vi "TranslateHom2D.vi"(0 "points":dbl[][](array[numeric])=[[0.0, 1.0, 79.632, 72.629, 0.0, 0.0, 1.0], [0.0, 2.0, 79.632, 159.629, 0.0, 0.0, 1.0], [0.0, 3.0, 90.632, 83.629, 0.0, 0.0, 1.0], [0.0, 4.0, 93.632, 156.629, 0.0, 0.0, 1.0], [0.0, 5.0, 192.632, 85.129, 0.0, 0.0, 1.0], [0.0, 6.0, 202.632, 159.629, 0.0, 0.0, 1.0], [0.0, 7.0, 208.632, 147.129, 0.0, 0.0, 1.0], [0.0, 8.0, 229.132, 68.129, 0.0, 0.0, 1.0], [0.0, 0.0, 0.0, 0.0, 0.0, 0.0, 0.0]], 1 "Camera":dbl[](array[numeric]), 2 "Robot":dbl[](array[numeric]), 5 "Steps":dbl[][](array[numeric])=[[0.0, 1.0, 79.632, 72.629, 0.0, 0.0, 1.0], [0.0, 2.0, 79.632, 159.629, 0.0, 0.0, 1.0], [0.0, 3.0, 90.632, 83.629, 0.0, 0.0, 1.0], [0.0, 4.0, 93.632, 156.629, 0.0, 0.0, 1.0], [0.0, 5.0, 192.632, 85.129, 0.0, 0.0, 1.0], [0.0, 6.0, 202.632, 159.629, 0.0, 0.0, 1.0], [0.0, 7.0, 208.632, 147.129, 0.0, 0.0, 1.0], [0.0, 8.0, 229.132, 68.129, 0.0, 0.0, 1.0], [0.0, 0.0, 0.0, 0.0, 0.0, 0.0, 0.0]], 9 "Angle":dbl, 11 "错误输入（无错误）":errorcluster, 12 "RealCamera":cluster{"X":dbl, "Y":dbl} {"X" format="%#_13g"}) -> (4 "ListPoints":dbl[][](array[numeric]), 6 "StringPoints":string[][](array[string]), 15 "错误输出":errorcluster)   [LabVIEW 2016]
uses:
  X86/halcondotnet.dll
panel:
  out "数组 2":dbl[](array[numeric])
  out "数组":dbl[](array[numeric])
  out "x-y":dbl
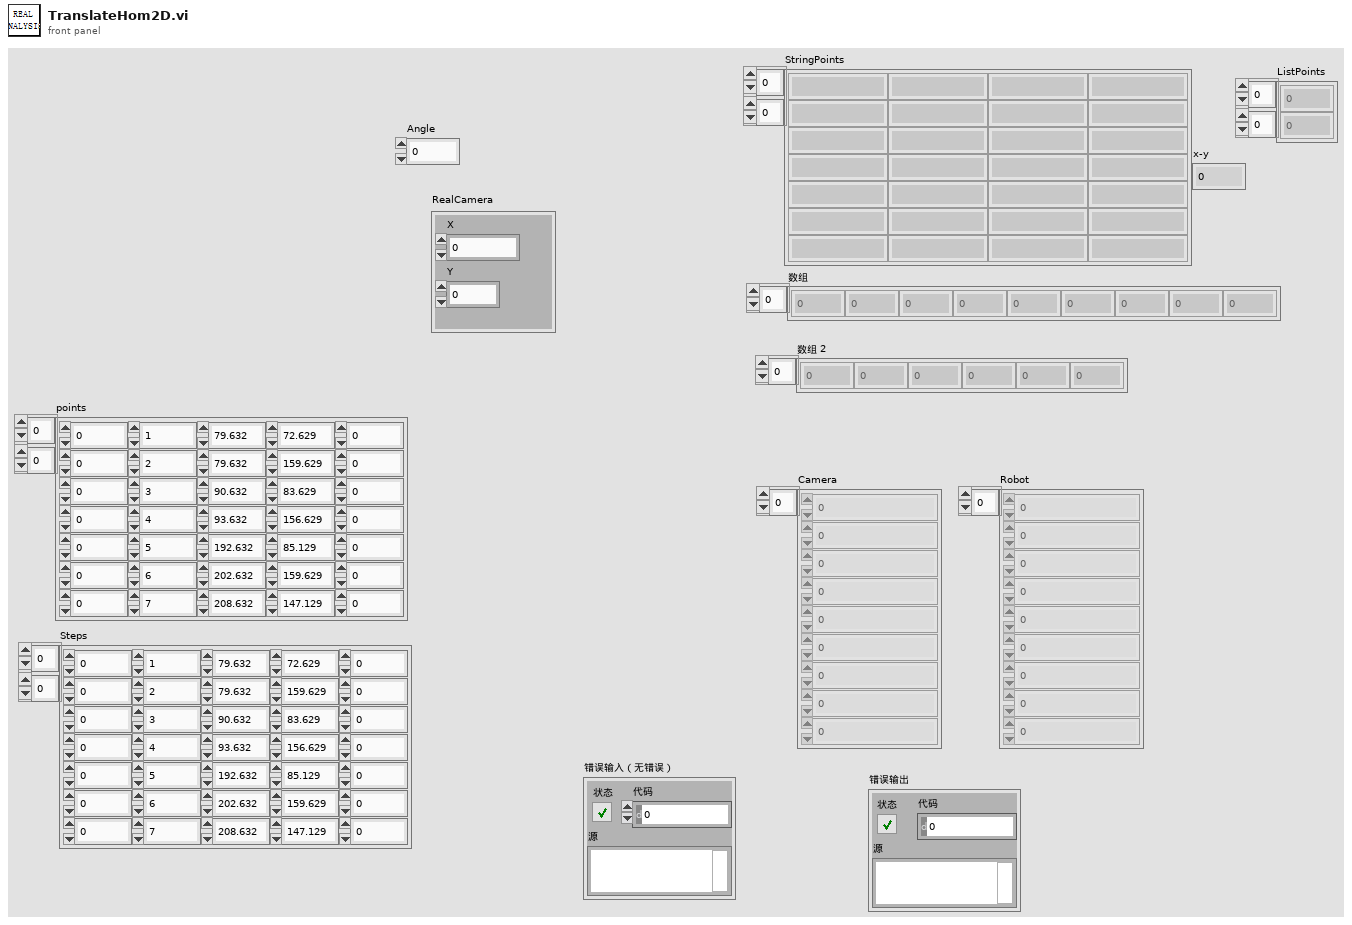
[diagram p1: front panel]
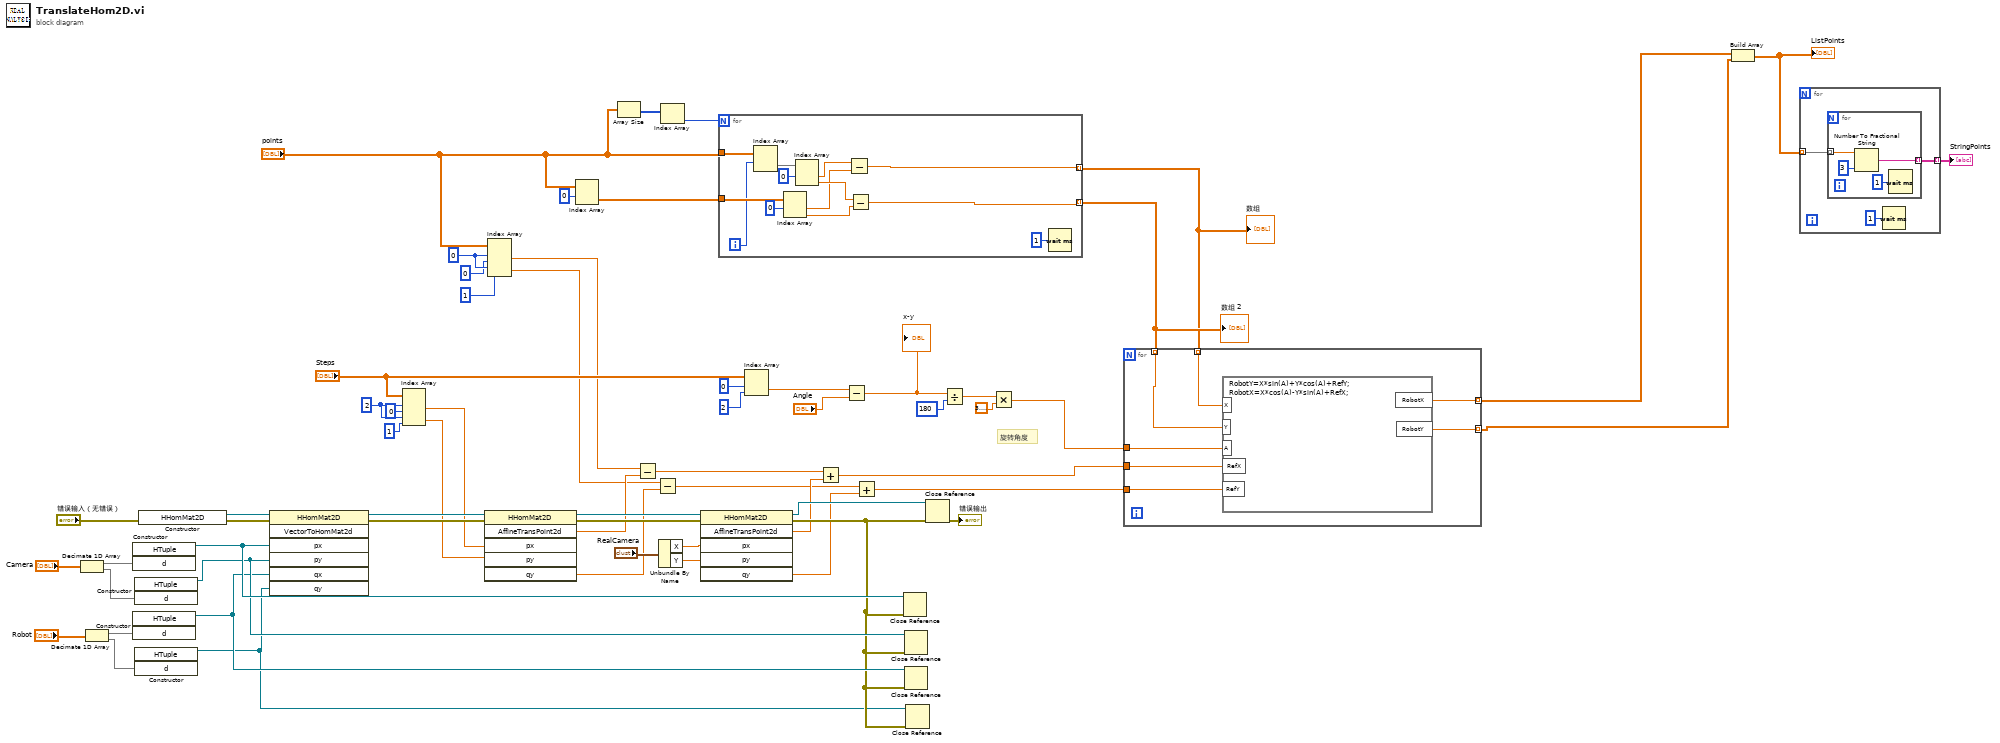
[diagram p0: block diagram]
diagram:
  w19 = 0 ("索引 (行)")
  w25 = 2 ("索引 (行)")
  # "旋转角度"
  n1 = Decimate 1D Array("Camera") -> (w60:dbl[], w59:dbl[])
  n2 = Decimate 1D Array("Robot") -> (w58:dbl[], w57:dbl[])
  n3 = constructor class="HTuple"("d"=w60) -> (reference out=w50:refnum<k24>)  [unwired: 3 in, 3 out]
  n4 = constructor class="HTuple"("d"=w58) -> (reference out=w48:refnum<k24>)  [unwired: 3 in, 3 out]
  n5 = constructor class="HTuple"("d"=w59) -> (reference out=w49:refnum<k24>)  [unwired: 3 in, 3 out]
  n6 = constructor class="HTuple"("d"=w57) -> (reference out=w46:refnum<k24>)  [unwired: 3 in, 3 out]
  n7 = constructor class="HHomMat2D"(error in="错误输入（无错误）") -> (reference out=w62:refnum<k24>, error out=w54:errorcluster)  [unwired: 2 in, 1 out]
  n8 = invoke class="HHomMat2D" method="VectorToHomMat2d"(reference=w62, error in=w54, "px"=w50, "py"=w49, "qx"=w48, "qy"=w46) -> (reference out=w61:refnum<k24>, error out=w53:errorcluster)  [unwired: 1 in, 5 out]
  n9 = Index Array(array="Steps", index (row) #1=w25, index (col) #1=0 ("禁用的索引 (列)"), index (row) #2=w25, index (col) #2=1 ("禁用的索引 (列)")) -> (element #1=w22:dbl, element #2=w21:dbl)
  n10 = invoke class="HHomMat2D" method="AffineTransPoint2d"(reference=w61, error in=w53, "px"=w22, "py"=w21) -> (reference out=w55:refnum<k24>, error out=w52:errorcluster, "AffineTransPoint2d"=w36:dbl, "qy"=w35:dbl)  [unwired: 2 in, 2 out]
  n11 = Index Array(array="points", index (row) #1=w19, index (col) #1=0 ("索引 (行)"), index (row) #2=w19, index (col) #2=1 ("索引 (行)")) -> (element #1=w16:dbl, element #2=w15:dbl)
  n12 = Index Array(array="points", index (row)=0 ("索引 (行)")) -> (element=w30:dbl[])  [unwired: 1 in]
  n13 = Array Size(array="points") -> (size(s)=w45:i32[])
  n14 = Subtract(x=w16, y=w36) -> (x-y=w32:dbl)
  n15 = Subtract(x=w15, y=w35) -> (x-y=w31:dbl)
  n16 = Unbundle By Name("RealCamera") -> ("X"=w39:dbl, "Y"=w38:dbl)
  n17 = Index Array(array=w45) -> (element=w44:i32)  [unwired: 1 in]
  n18 = invoke class="HHomMat2D" method="AffineTransPoint2d"(reference=w55, error in=w52, "px"=w39, "py"=w38) -> (reference out=w51:refnum<k24>, error out=w47:errorcluster, "AffineTransPoint2d"=w34:dbl, "qy"=w33:dbl)  [unwired: 2 in, 2 out]
  n19 = for {
    N: w44 -> [_]
    tunnel: w30 -> [w75]
    tunnel: "points" -> [w72]
    tunnel: [w64] -> w8 mode=indexing
    tunnel: [w63] -> w43 mode=indexing
    i -> [w65]
    n20 = Index Array(array=w72, index (row)=w65) -> (element=w73:dbl[])  [unwired: 1 in]
    n21 = Index Array(array=w75, index #1=0 ("索引")) -> (element #1=w67:dbl, element #2=w69:dbl)  [unwired: 1 in]
    n22 = Index Array(array=w73, index #1=0 ("索引")) -> (element #1=w68:dbl, element #2=w70:dbl)  [unwired: 1 in]
    n23 = Subtract(x=w68, y=w67) -> (x-y=w64:dbl)
    n24 = Subtract(x=w70, y=w69) -> (x-y=w63:dbl)
    n25 = Wait (ms)(milliseconds to wait=u32 1 ("等待时间（毫秒）")) -> ()  [unwired: 1 out]
  }
  "数组" <- w8
  "数组 2" <- w43
  n26 = Index Array(array="Steps", index (row)=0 ("索引 (行)"), index (col)=2 ("索引 (行)")) -> (element=w7:dbl)
  n27 = Add(x=w32, y=w34) -> (x+y=w10:dbl)
  n28 = Subtract(x=w7, y="Angle") -> (x-y=w5:dbl)
  "x-y" <- w5
  n29 = Add(x=w31, y=w33) -> (x+y=w11:dbl)
  n30 = Close Reference(reference=w50, error in (no error)=w47) -> ()  [unwired: 1 out]
  n31 = Close Reference(reference=w49, error in (no error)=w47) -> ()  [unwired: 1 out]
  n32 = Close Reference(reference=w48, error in (no error)=w47) -> ()  [unwired: 1 out]
  n33 = Close Reference(reference=w46, error in (no error)=w47) -> ()  [unwired: 1 out]
  n34 = Close Reference(reference=w51, error in (no error)=w47) -> (error out=→"错误输出":errorcluster)
  n35 = Divide(x=w5, y=180) -> (x/y=w3:dbl)
  n36 = Multiply(x=w3, y=3.141592653589793) -> (x*y=w1:dbl)
  n37 = for {
    tunnel: w8 -> [w77] mode=indexing
    tunnel: w43 -> [w76] mode=indexing
    tunnel: w10 -> [w82]
    tunnel: w11 -> [w81]
    tunnel: w1 -> [w80]
    tunnel: [w79] -> w14 mode=indexing
    tunnel: [w78] -> w13 mode=indexing
    n38 = formula code="RobotY=X*sin(A)+Y*cos(A)+RefY;\nRobotX=X*cos(A)-Y*sin(A)+RefX;"("X"=w77, "Y"=w76, "RefX"=w82, "RefY"=w81, "A"=w80) -> ("RobotX"=w79:dbl, "RobotY"=w78:dbl)
  }
  n39 = Build Array(w14, w13) -> (w12:dbl[][])
  "ListPoints" <- w12
  n40 = for {
    tunnel: w12 -> [w85] mode=indexing
    tunnel: [w84] -> w41 mode=indexing
    n41 = for {
      tunnel: w85 -> [w89] mode=indexing
      tunnel: [w88] -> w84 mode=indexing
      n42 = Number To Fractional String(number=w89, precision (6)=i16 3 ("精度(6)")) -> (F-format string=w88:string)  [unwired: 2 in]
      n43 = Wait (ms)(milliseconds to wait=u32 1 ("等待时间（毫秒）")) -> ()  [unwired: 1 out]
    }
    n44 = Wait (ms)(milliseconds to wait=u32 1 ("等待时间（毫秒）")) -> ()  [unwired: 1 out]
  }
  "StringPoints" <- w41
